vi "uMsg Detach Payload.vi"(8 "error in (no error)":errorcluster, 11 "uMsg in":refnum<class "uMsg.lvclass">) -> (0 "error out":errorcluster, 1 "payload":refnum<class "uData.lvclass">, 2 "uMsg headers":refnum<class "uMsg.lvclass">)   [LabVIEW 2023, in "uLib.lvlib" / "uMsg.lvclass"]
doc: "Detach the payload from the message. The output is a message with only headers and metadata.\nThe payload object is returned separately.\nThis is to improve resource efficiency if handling large sets of data, in which case the payload is not duplicated when requiring a copy of the headers and metadata like the timestamp."
uses:
  uMsg.lvclass
  uData/uData/uData.lvclass
  uMsg.lvclass/uMsg.ctl
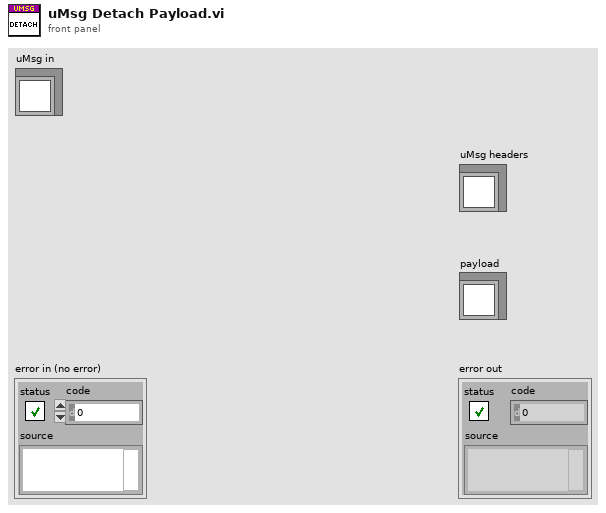
[diagram p1: front panel]
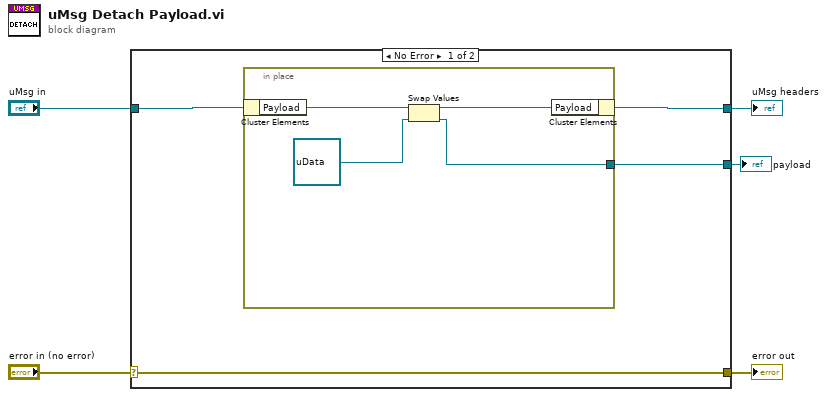
[diagram p0: block diagram]
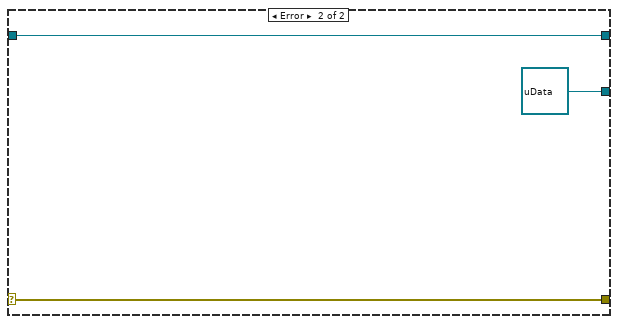
[diagram p2: hidden frame]
diagram:
  n1 = case shown="No Error" "error in (no error)" {
    selector: "error in (no error)" -> [w9 w16]
    tunnel: [w9 w16] -> w4
    tunnel: [w7 w15] -> w2
    tunnel: "uMsg in" -> [w8 w15]
    tunnel: [w6 refnum<class "uData.lvclass"> refnum ("uData.lvlib:uData.lvclass")] -> w1
    frame No Error {
      n2 = in-place {
        in-place-border: [w10] -> w6
        n3 = in-place-cluster #1(w8) -> ("Payload"=w13:refnum<class "uData.lvclass">)
        n4 = Swap Values(12:w13, 14:refnum<class "uData.lvclass"> refnum ("Payload")) -> (1:w11:refnum<class "uData.lvclass">, 3:w10:refnum<class "uData.lvclass">)  [unwired: 1 in]
        n5 = in-place-cluster #1("Payload"=w11) -> (w7:refnum<class "uMsg.lvclass">)
      }
    }
    frame Error {
    }
  }
  "error out" <- w4
  "uMsg headers" <- w2
  "payload" <- w1
